vi "Initialize LTI ULS.vi"(8 "error in (no error)":errorcluster, 10 "COM Port":refnum<visa-resource-name>, 11 "MWWL Verification in":refnum<class "MWWL Verification.lvclass">) -> (0 "error out":errorcluster, 3 "MWWL Verification out":refnum<class "MWWL Verification.lvclass">)   [LabVIEW 2017, in "MWWL Verification.lvlib" / "MWWL Verification.lvclass"]
uses:
  MWWL Verification.lvclass
  LTI ULS Actor/LTI ULS Actor.lvclass
  <vilib>/ActorFramework/Actor/Actor.lvclass
  Sensor Actor/Sensor Messages/Set Sensor COM Port Msg/Set Sensor COM Port Msg.lvclass
  LTI ULS Actor/LTI ULS Actor Messages/Configure LTI ULS Msg/Configure LTI ULS Msg.lvclass
  C:/Users/dev/Documents/CODE/LabVIEW/microwaveverify/trunk/MWWL Verification/Sensor Actor/Sensor/Sensor.lvclass
  C:/Users/dev/Documents/CODE/LabVIEW/microwaveverify/trunk/MWWL Verification/Actor Monitor/Actor/Monitored Actor.lvclass
  C:/Program Files (x86)/National Instruments/LabVIEW 2017/vi.lib/ActorFramework/Actor/Actor.lvclass
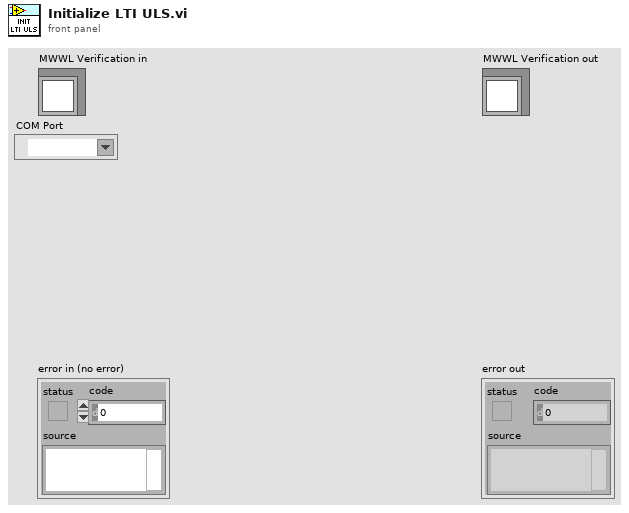
[diagram p1: front panel]
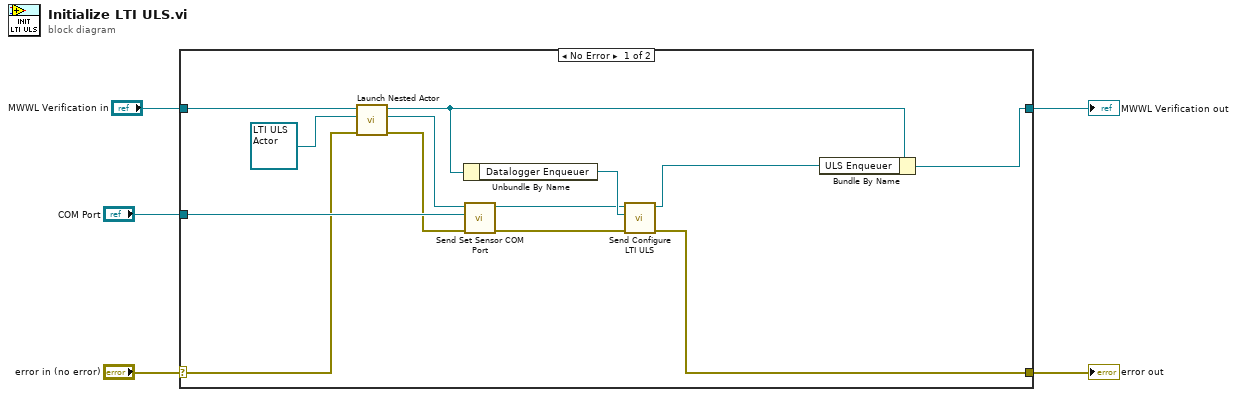
[diagram p0: block diagram]
diagram:
  n1 = case shown="No Error" "error in (no error)" {
    selector: "error in (no error)" -> [w10 w20]
    tunnel: [w9 w20] -> w4
    tunnel: [w7 w19] -> w2
    tunnel: "MWWL Verification in" -> [w18 w19]
    tunnel: "COM Port" -> [w15 _]
    frame No Error {
      n2 = call <vilib>:"Launch Nested Actor.vi"("error in (no error)"=w10, "Nested Actor"=refnum<class "LTI ULS Actor.lvclass"> refnum ("LTI ULS.lvlib:LTI ULS Actor"), "Caller Actor in"=w18) -> ("error out"=w14:errorcluster, "Nested Actor's Enqueuer"=w16:refnum<class "Message Enqueuer.lvclass">, "Caller Actor out"=w8:refnum<class "MWWL Verification.lvclass">)  [unwired: 6 in]
      n3 = Unbundle By Name(w8) -> ("Datalogger Enqueuer"=w13:refnum<class "Message Enqueuer.lvclass">)
      n4 = call "Send Set Sensor COM Port.vi"("error in (no error)"=w14, "COM Port"=w15, "Message Enqueuer in"=w16) -> ("error out"=w11:errorcluster, "Message Enqueuer out"=w12:refnum<class "Message Enqueuer.lvclass">)  [unwired: 7 in]
      n5 = call "Send Configure LTI ULS.vi"("error in (no error)"=w11, "Datalogger Enqueuer"=w13, "Message Enqueuer in"=w12) -> ("error out"=w9:errorcluster, "Message Enqueuer out"=w6:refnum<class "Message Enqueuer.lvclass">)  [unwired: 7 in]
      n6 = Bundle By Name(cluster=w8, "ULS Enqueuer"=w6) -> (w7:refnum<class "MWWL Verification.lvclass">)
    }
    frame Error {
    }
  }
  "error out" <- w4
  "MWWL Verification out" <- w2
